vi "Write comand Stop read.vi"(8 "error in (no error)":errorcluster, 9 "Stop read":bool, 11 "VISA Refnum in":refnum<visa-resource-name>) -> (0 "error out":errorcluster, 3 "VISA Refnum out":refnum<visa-resource-name>)   [LabVIEW 2017, in "IL Driver Library.lvlib"]
uses:
  IL Driver library.lvlib
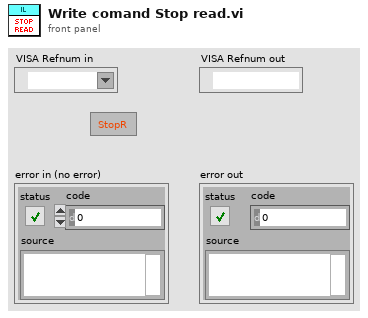
[diagram p1: front panel]
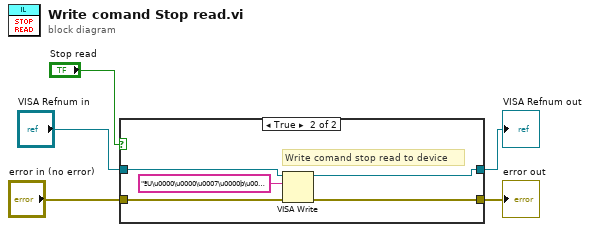
[diagram p0: block diagram]
diagram:
  n1 = case shown="True" "Stop read" {
    tunnel: "VISA Refnum in" -> [w7 w11]
    tunnel: "error in (no error)" -> [w6 w10]
    tunnel: [w7 w9] -> w4
    tunnel: [w6 w8] -> w5
    frame False {
    }
    frame True {
      # "Write comand stop read to device"
      n2 = VISA Write(VISA resource name=w11, write buffer="ªU\u0000\u0000\u0007\u0000þ\u0005\u0001", error in (no error)=w10) -> (VISA resource name out=w9:refnum<visa-resource-name>, error out=w8:errorcluster)  [unwired: 1 out]
    }
  }
  "error out" <- w5
  "VISA Refnum out" <- w4
